vi "Inititializing.vi"(11 "Parameters":T3={"Mass"=6.0, "GearRatio"=25.0, "Radius"=0.015, "Resistance"=0.089, "Ki"=0.0053, "Ke"=0.0061, "Friction"=0.0}) -> (3 "Plant":T2)   [LabVIEW 2017]
uses:
  <vilib>/Analysis/Matrix/Datatypes/RealMatrix.ctl
  <vilib>/Analysis/Matrix/Datatypes/ComplexMatrix.ctl
  <vilib>/Analysis/Matrix/NI_Matrix.lvlib
panel:
  in  "Poles":T4=[[-10.0+0.0i], [-7.0+0.0i]]
  in  "Plant":T2={"Gains"={"A"=[[0.0, 1.0], [0.0, -166.98]], "B"=[[0.0], [16.43]], "C"=[[1.0, 0.0]], "D"=[[0.0]], "Q"=[[0.0, 0.0], [0.0, 0.0]], "R"=[[0.005]], "K"=[], "Kff"=[], "L"=[[0.001], [1e-06]]}, "X"=[[0.0], [0.0]]}
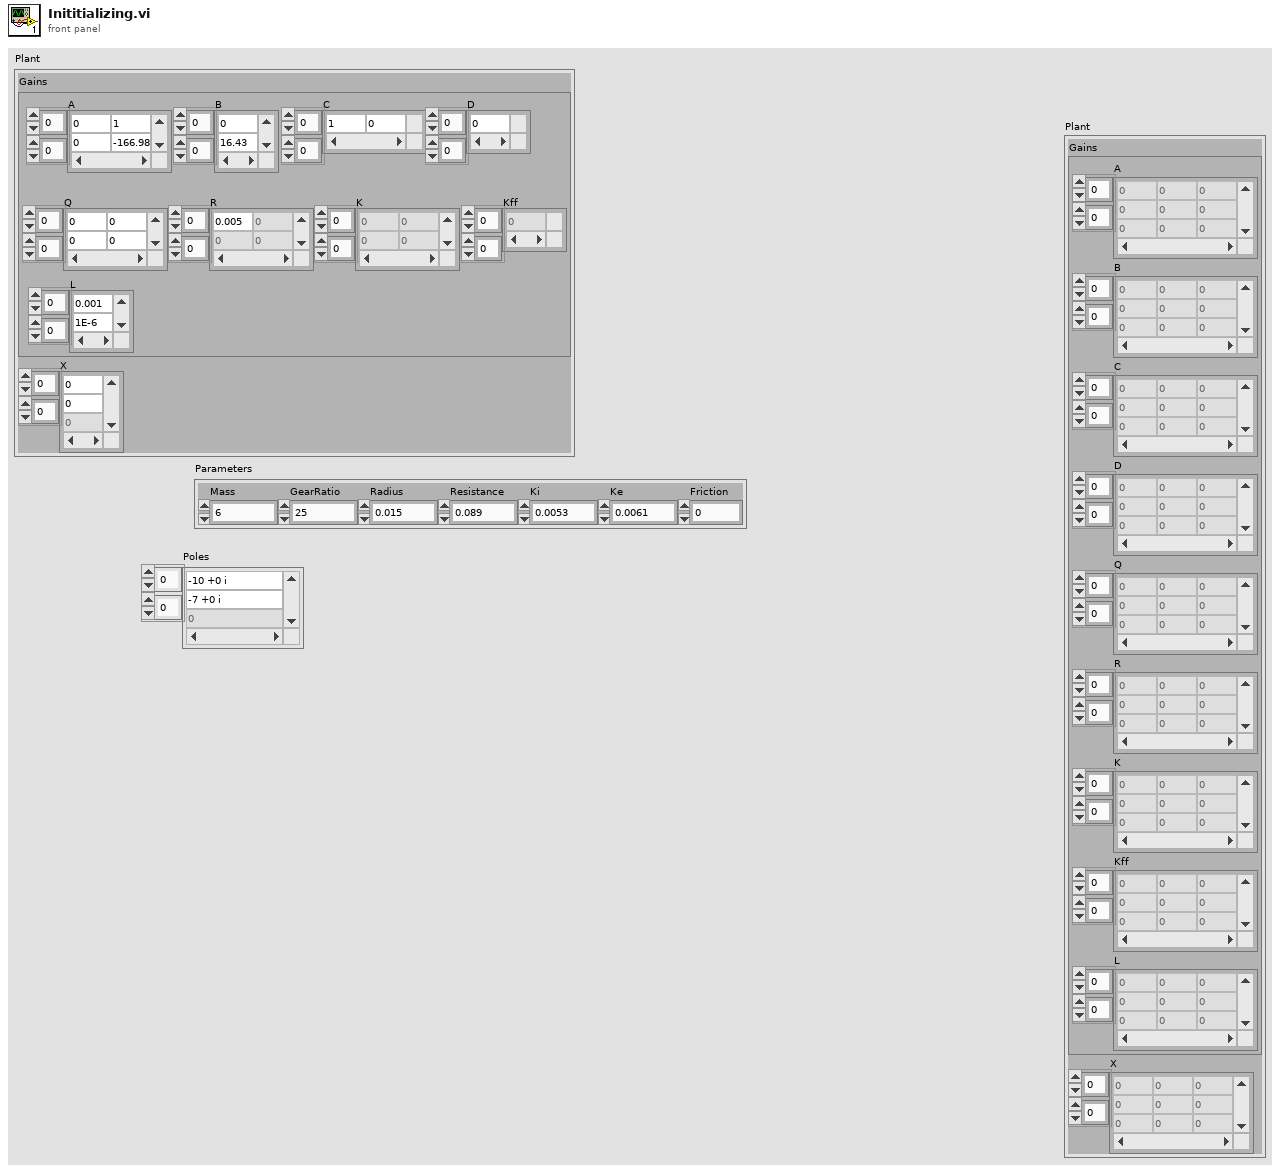
[diagram p1: front panel]
types:
  T1 = typedef "NI_Matrix.lvlib/RealMatrix.ctl" = dbl[][]
  T2 = cluster{"Gains":cluster{"A":T1, "B":T1, "C":T1, "D":T1, "Q":T1, "R":T1, "K":T1, "Kff":T1, "L":T1}, "X":T1}
  T3 = cluster{"Mass":dbl, "GearRatio":dbl, "Radius":dbl, "Resistance":dbl, "Ki":dbl, "Ke":dbl, "Friction":dbl}
  T4 = typedef "NI_Matrix.lvlib/ComplexMatrix.ctl" = cdb[][]
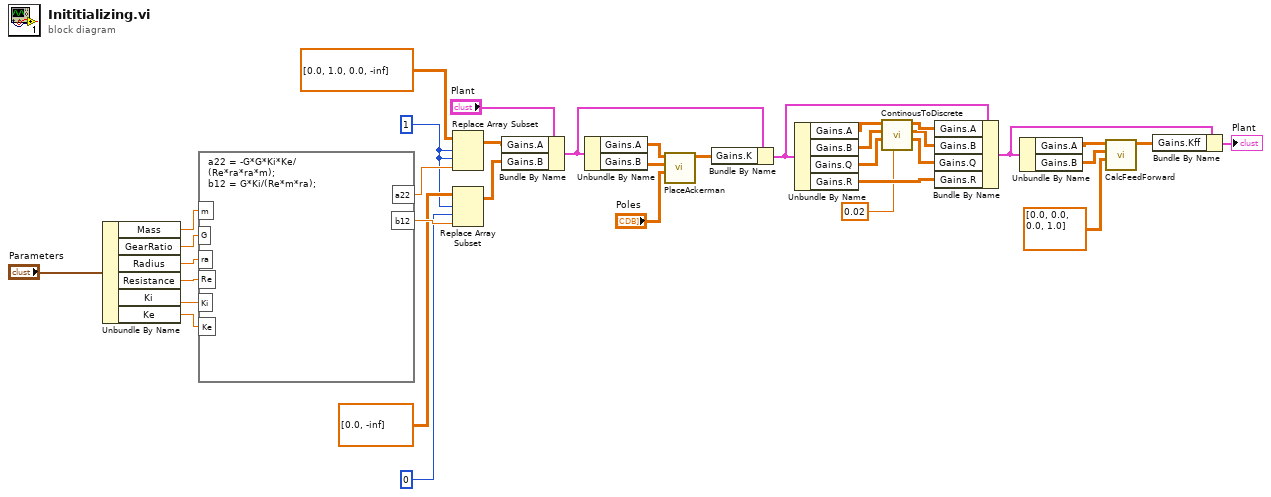
[diagram p0: block diagram]
diagram:
  w7 = 1 ("index (col)")
  n1 = Unbundle By Name("Parameters") -> ("Mass"=w18:dbl, "GearRatio"=w17:dbl, "Radius"=w16:dbl, "Resistance"=w15:dbl, "Ki"=w14:dbl, "Ke"=w13:dbl)
  n2 = formula code="a22 = -G*G*Ki*Ke/\n(Re*ra*ra*m);\nb12 = G*Ki/(Re*m*ra);"("m"=w18, "G"=w17, "ra"=w16, "Ki"=w14, "Re"=w15, "Ke"=w13) -> ("a22"=w12:dbl, "b12"=w11:dbl)
  n3 = Replace Array Subset(array=T1 [[0.0, 1.0], [0.0, -inf]] ("matrix"), new element=w12, index (row)=w7, index (col)=w7) -> (w6:T1)
  n4 = Replace Array Subset(array=T1 [[0.0], [-inf]] ("matrix"), new element=w11, index (row)=w7, index (col)=0 ("disabled index (row)")) -> (w5:T1)
  n5 = Bundle By Name(cluster="Plant", "Gains.A"=w6, "Gains.B"=w5) -> (w1:T2)
  n6 = Unbundle By Name(w1) -> ("Gains.A"=w30:T1, "Gains.B"=w29:T1)
  n7 = call "PlaceAckerman.vi"("Poles"="Poles", "B"=w29, "A"=w30) -> ("K"=w21:T1)  [unwired: 8 in]
  n8 = Bundle By Name(cluster=w1, "Gains.K"=w21) -> (w27:T2)
  n9 = Unbundle By Name(w27) -> ("Gains.A"=w36:T1, "Gains.B"=w35:T1, "Gains.Q"=w26:T1, "Gains.R"=w24:T1)
  n10 = call "ContinousToDiscrete.vi"("dt"=0.02, "Q"=w26, "B"=w35, "A"=w36) -> ("Q_d"=w25:T1, "B_d"=w33:T1, "A_d"=w34:T1)  [unwired: 4 in, 1 out]
  n11 = Bundle By Name(cluster=w27, "Gains.A"=w34, "Gains.B"=w33, "Gains.Q"=w25, "Gains.R"=w24) -> (w20:T2)
  n12 = Unbundle By Name(w20) -> ("Gains.A"=w23:T1, "Gains.B"=w32:T1)
  n13 = call "CalcFeedForward.vi"("Q"=T1 [[0.0, 0.0], [0.0, 1.0]], "B"=w32, "A"=w23) -> ("Kff"=w31:T1)  [unwired: 8 in]
  n14 = Bundle By Name(cluster=w20, "Gains.Kff"=w31) -> (→"Plant":T2)
